vi "String_Bool to (0,1)String.vi"(4 "in":bool) -> (1 "0,1 string":string)   [LabVIEW 2015]
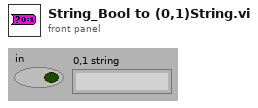
[diagram p1: front panel]
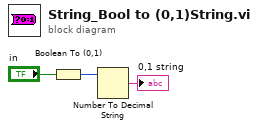
[diagram p0: block diagram]
diagram:
  n1 = Boolean To (0,1)(Boolean="in") -> (0, 1=w3:i16)
  n2 = Number To Decimal String(number=w3) -> (decimal integer string=→"0,1 string":string)  [unwired: 1 in]
